vi "Main.vi"() -> ()   [LabVIEW 2020]
doc: "Cet exemple de projet Mesure continue est basé sur le modèle Gestionnaire de messages dans une file d'attente.\n\nLa boucle de gestion d'événements génère des messages en fonction des actions sur l'interface utilisateur.\n\nLa boucle de gestion de messages traite les messages générés par la boucle de gestion d'événements ou par d'autres messages. Il y a aussi des sous-VIs de boucle de gestion de messages d'acquisition et d'enregistrement, ainsi qu'une boucle de mise à jour du graphe déroulant."
uses:
  Settings/Settings.ctl
  Acquisition/Hardware Configuration.ctl
  Acquisition/Signal Type.ctl
  Logging/Logging Configuration.ctl
  controls/UI Data.ctl
  controls/UI State.ctl
  support/Message Queue/Enqueue Message (Single).vi
  support/Message Queue/Enqueue Message (Array).vi
  <vilib>/Utility/error.llb/Error Cluster From Error Code.vi
  <vilib>/ErrorRing/Error Ring.xnode
  Acquisition/Acquisition.lvlib
  Logging/Logging.lvlib
  Settings/Settings.lvlib
  support/User Event - Stop/User Event - Stop.lvlib
  support/Message Queue/Message Queue.lvlib
  Settings/Settings Dialog.vi
panel:
  in  "Panneaux":T1(tab)
  in  "Param status":bool
  out "Données":waveform(dbl)[](graph)
  out "État":string
  in  "Quitter":bool
  in  "Arrêter":bool
  in  "Démarrer":bool
  in  "Paramètres":bool
  out "Valeur des thermistantes 2":dbl[](array[numeric])
  out "Valeur des thermistantes":dbl[](array[numeric])
  # "TODO:\n\n- Mettre le port des paramètres pour connection\n- Faire entrer les param dans la boucle d'affichage\n- Valider l'enregistrement  du data\n- Faire sous-vi ordre 0\n- Faire sous-vi ordre 1"
  # "MAPA Tech"
  # "MAPA Tech"
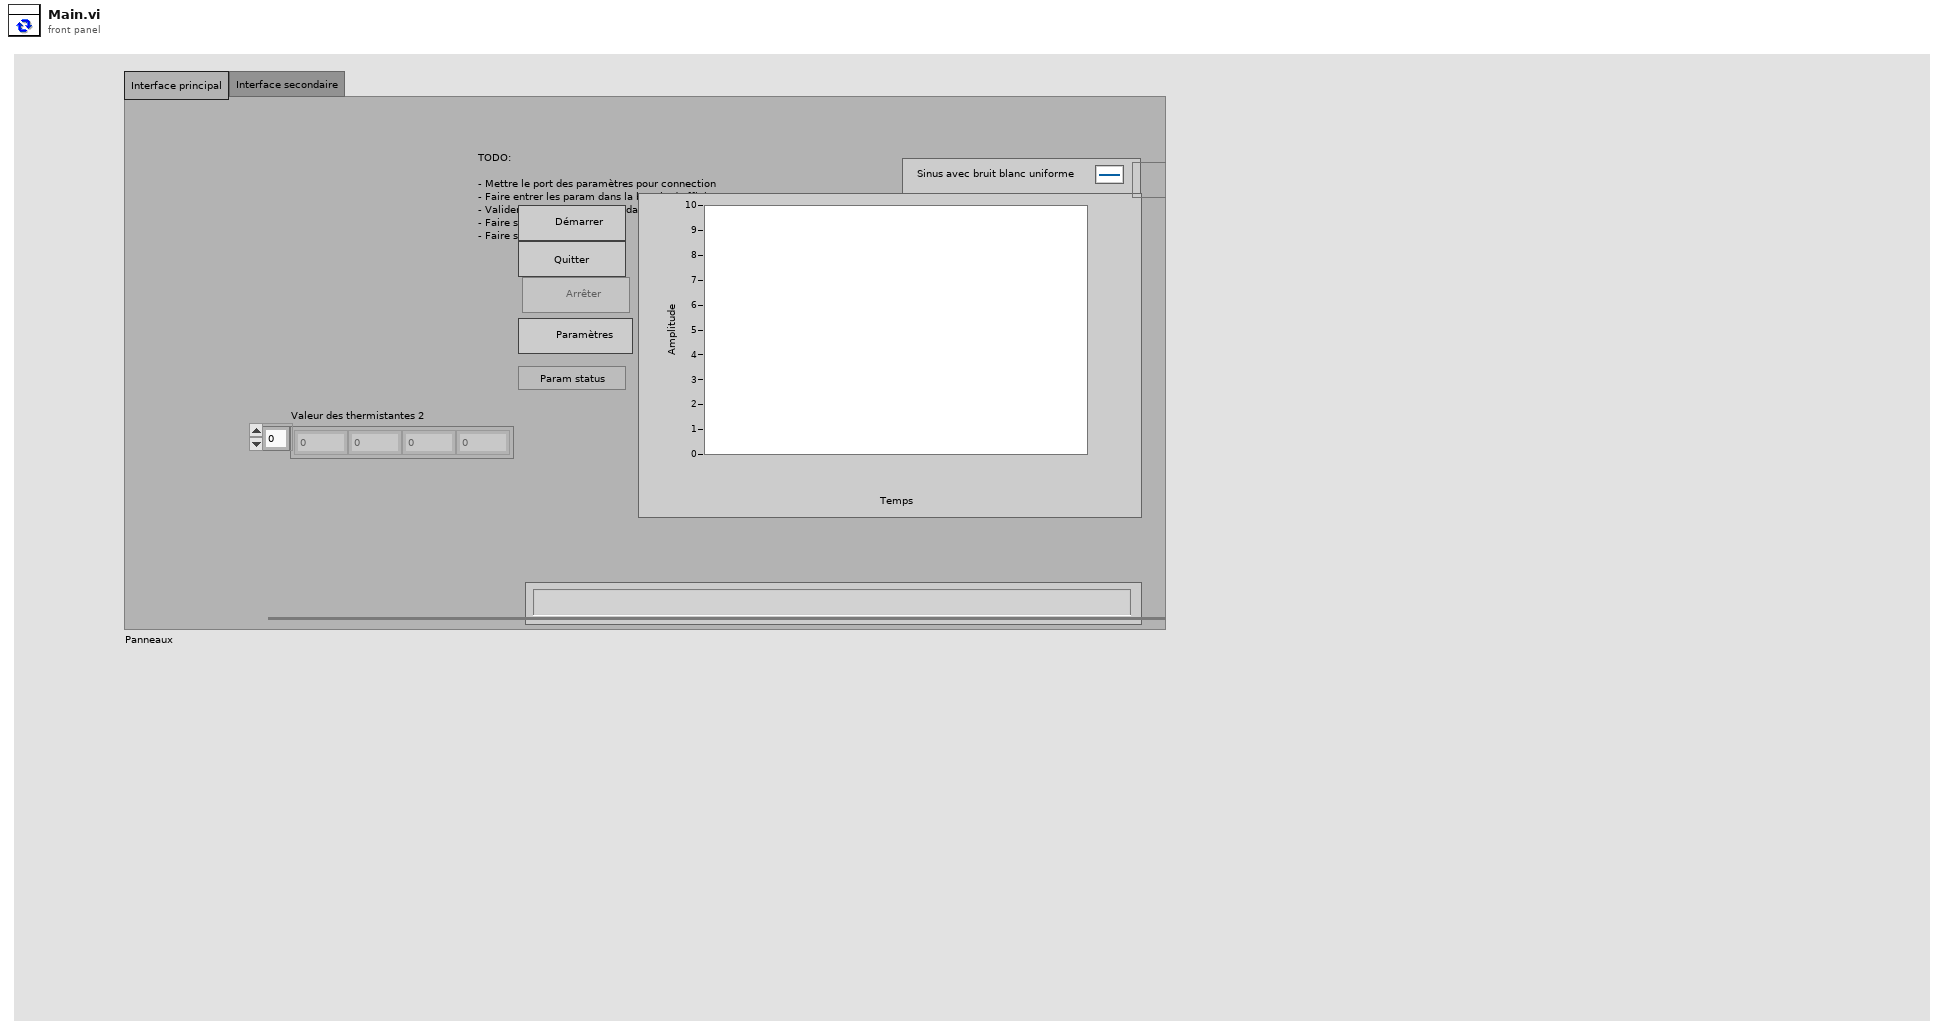
[diagram p1: front panel]
types:
  T1 = enum32{"Interface principal", "Interface secondaire"}
  T2 = typedef "UI State.ctl" = enum16{"Idle", "Acquiring and Logging", "Waiting for Exit", "Waiting for Exit (Acq Stopped)", "Waiting for Exit (Log Stopped)", "Waiting for Stop", "Waiting for Stop (Acq Stopped)", "Waiting for Stop (Log Stopped)"}
  T3 = typedef "UI Data.ctl" = cluster{"Réf. de Démarrer":refnum<vi>, "Réf. d'Arrêter":refnum<vi>, "Réf. de Paramètres":refnum<vi>, "Réf. de Quitter":refnum<vi>, "Réf. d'état":refnum<vi>, "Réf. de données":refnum<vi>, "Ref. Moyennage sélectionneur":refnum<vi>, "Ref. Param status":refnum<vi>}
  T4 = typedef "Settings.lvlib/Settings.ctl" = cluster{"Configuration du matériel":T5, "Configuration de l'enregistrement":T7, "Mode de longueur d'onde":cluster{"Choix du mode":bool, "Commande numérique":dbl}, "périphérique":cluster{"Nom du périphérique":tag}}
  T5 = typedef "Acquisition.lvlib/Hardware Configuration.ctl" = cluster{"Refnum de matériel <À remplacer>":string, "Type de signal <À remplacer>":T6}
  T6 = typedef "Acquisition.lvlib/Signal Type.ctl" = enum16{"Sine Wave", "Square with Noise", "Signal triangulaire", "Simulation DAQ"}
  T7 = typedef "Logging.lvlib/Logging Configuration.ctl" = cluster{"Chemin de base du fichier journal":path, "Référence de fichier TDMS":refnum<k34>}
  T8 = cluster{"état":bool, "code":i32, "source":string}
  T9 = typedef "Message Queue.lvlib/All Message Queues.ctl" = cluster{"IU":refnum<queue>, "Acquisition":refnum<queue>, "Enregistrement":refnum<queue>}
  T10 = cluster{"Choix du mode":bool, "Commande numérique":dbl}
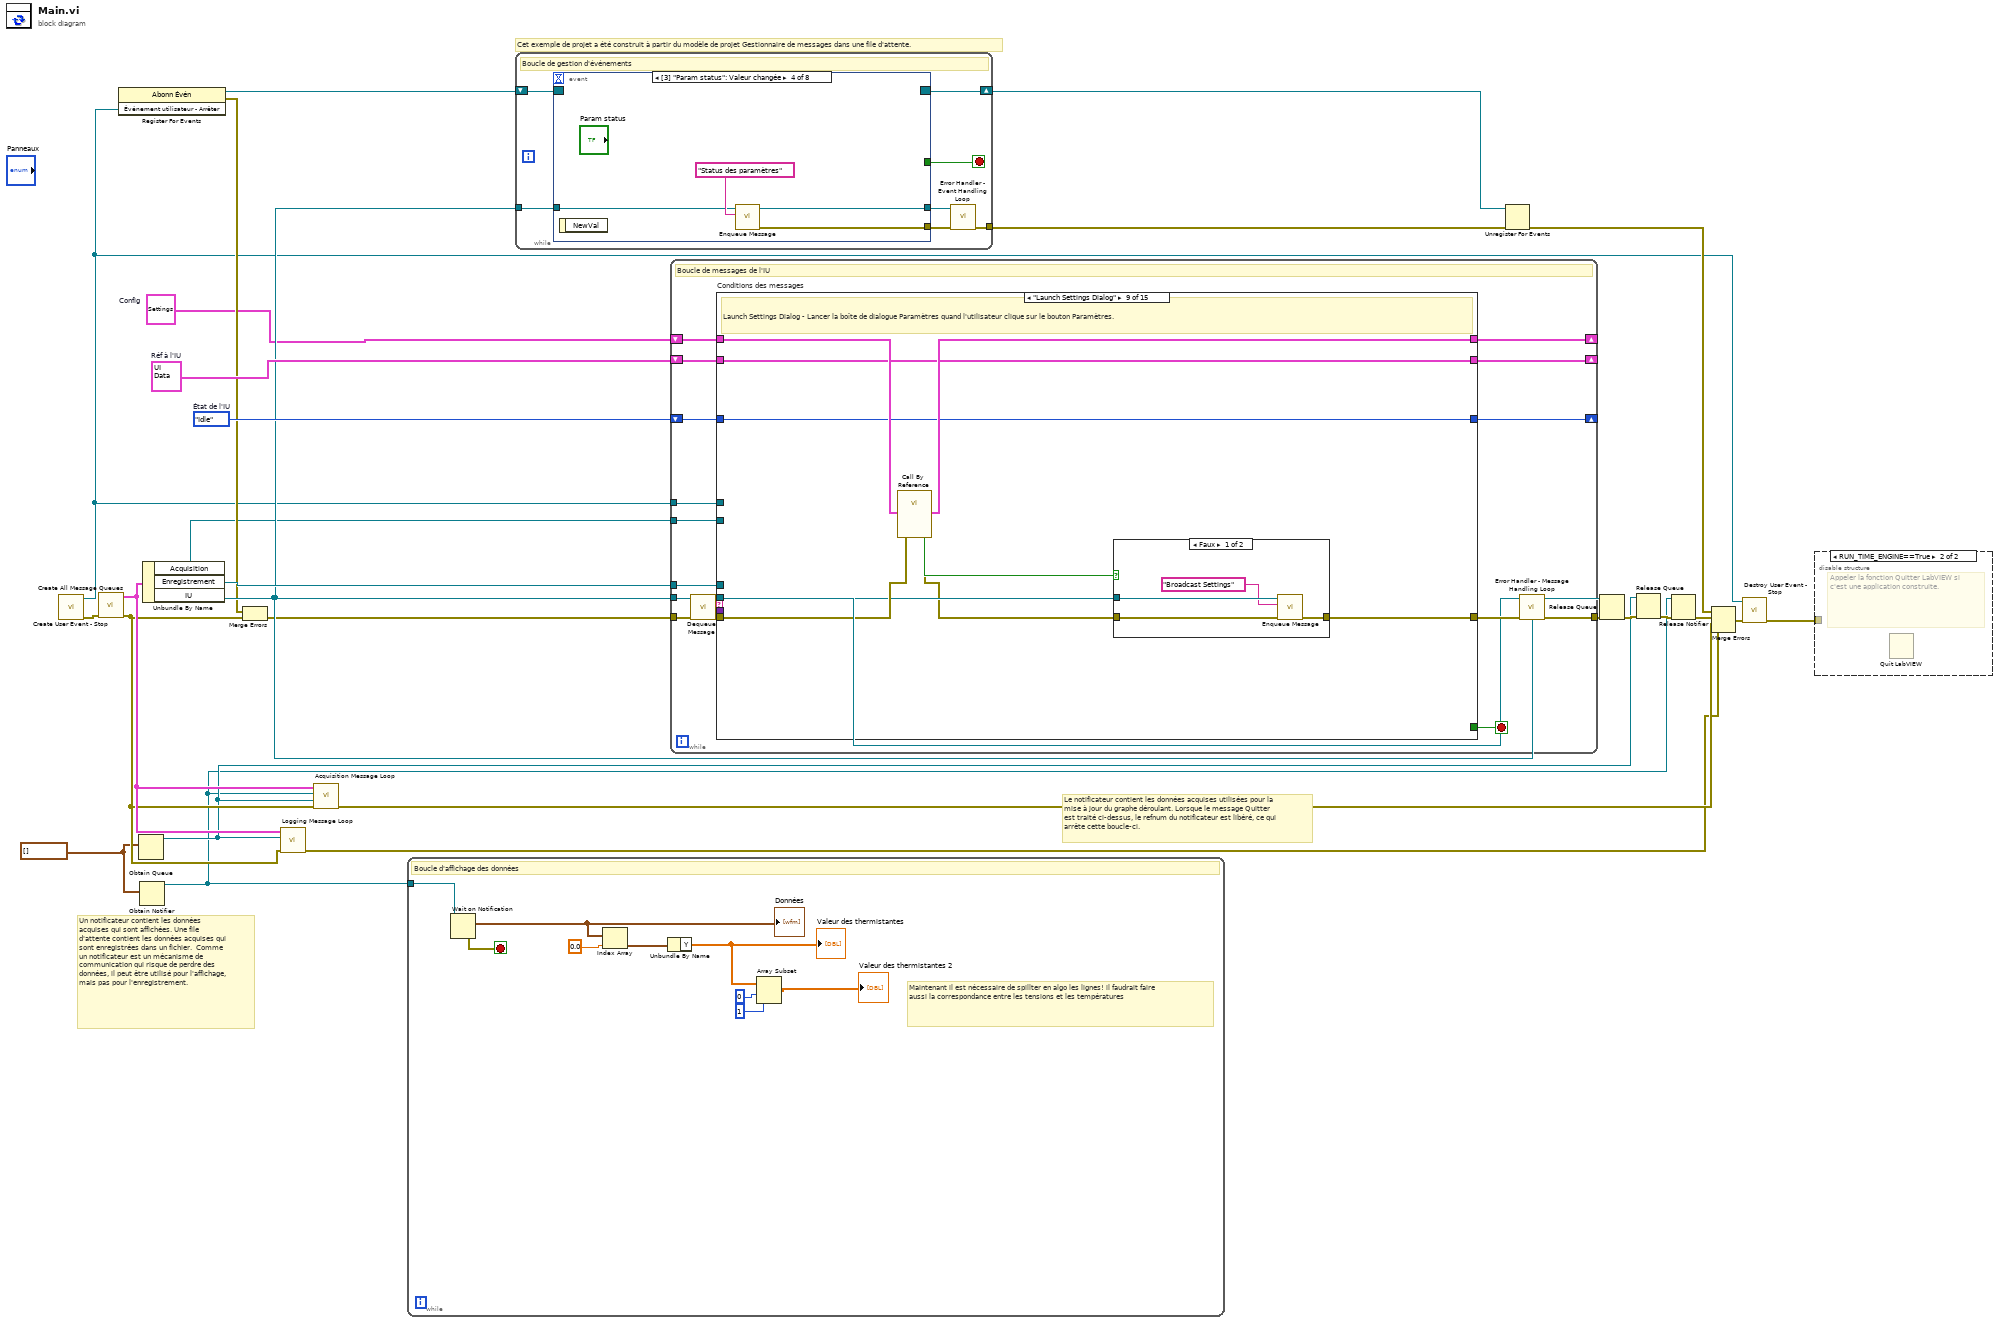
[diagram p0: block diagram]
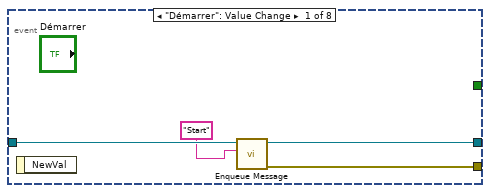
[diagram p3: hidden frame]
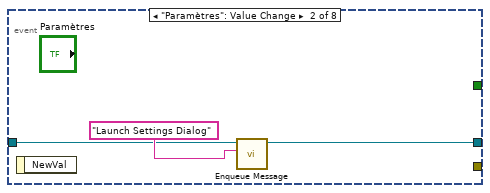
[diagram p4: hidden frame]
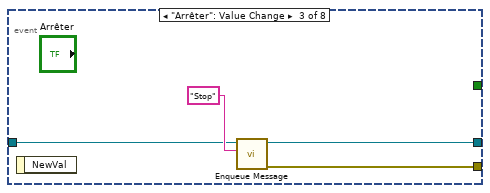
[diagram p5: hidden frame]
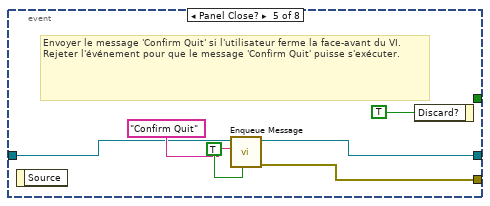
[diagram p6: hidden frame]
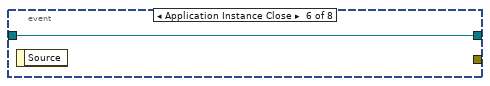
[diagram p7: hidden frame]
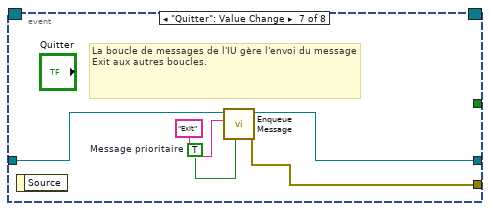
[diagram p8: hidden frame]
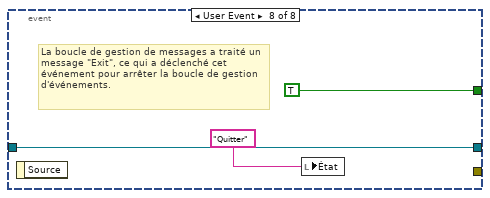
[diagram p9: hidden frame]
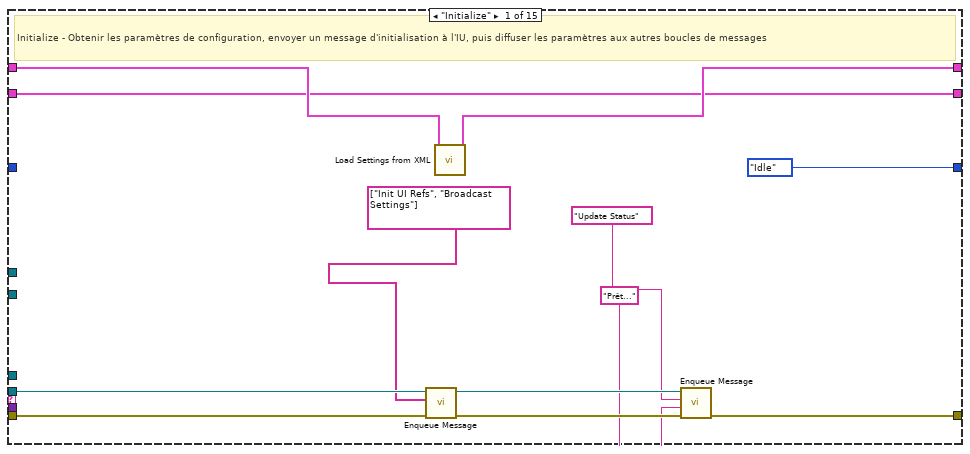
[diagram p10: hidden frame]
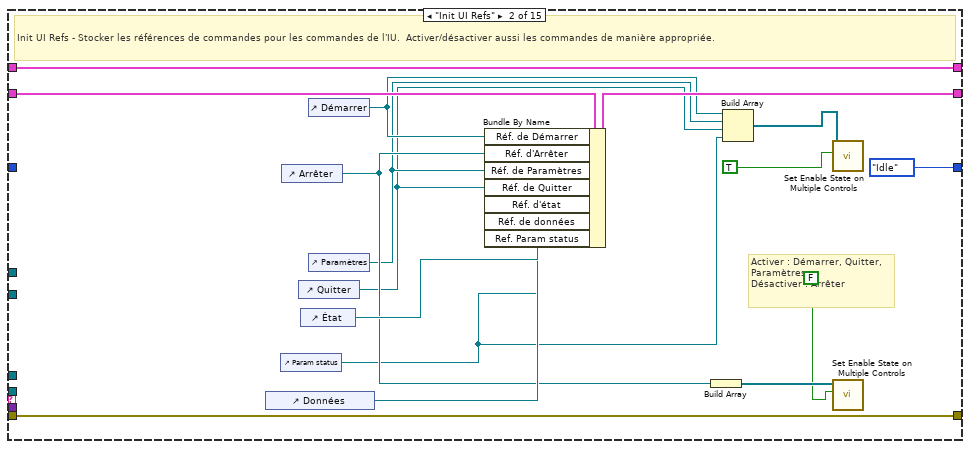
[diagram p11: hidden frame]
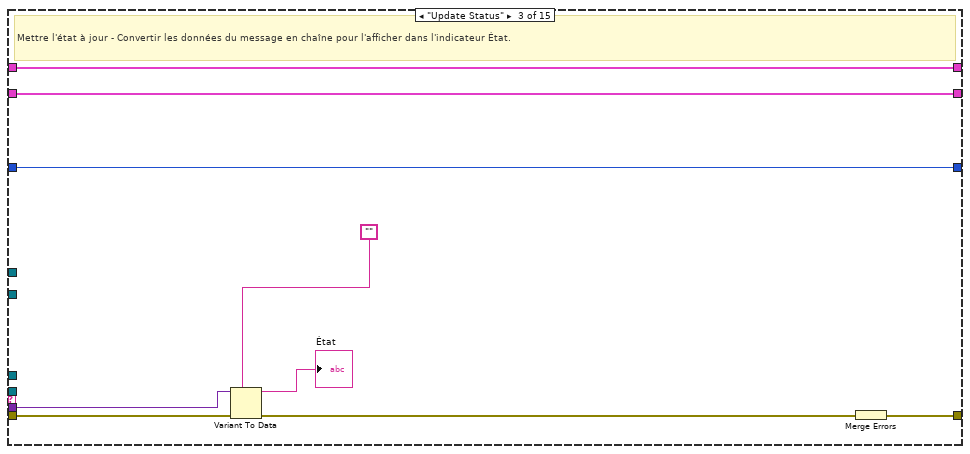
[diagram p12: hidden frame]
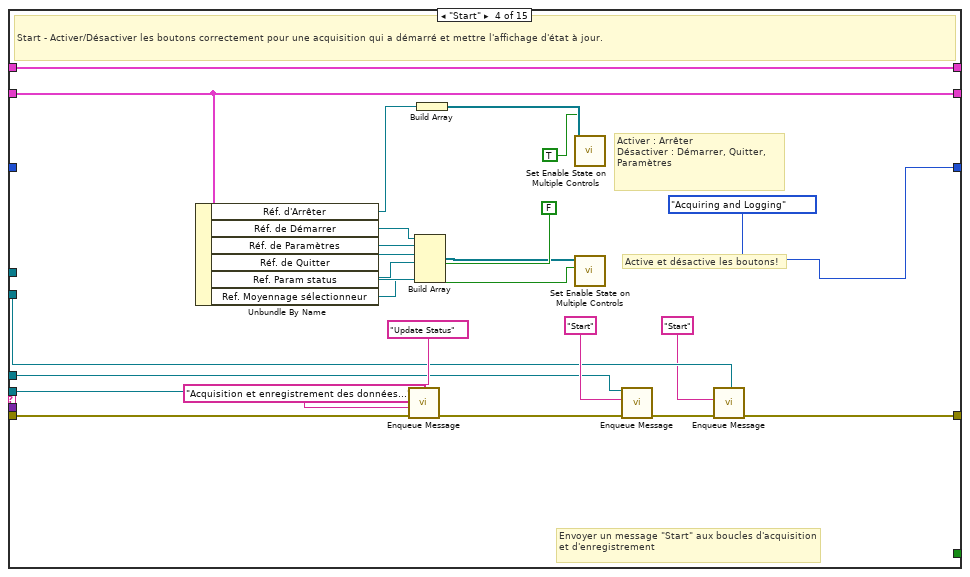
[diagram p13: hidden frame]
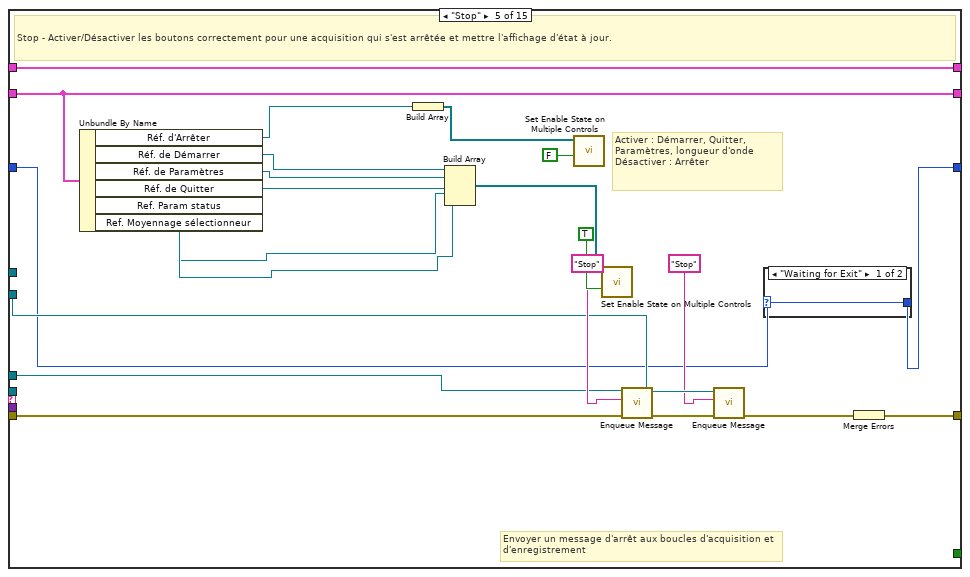
[diagram p14: hidden frame]
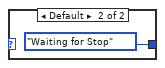
[diagram p15: hidden frame]
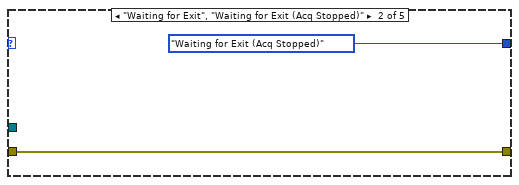
[diagram p17: hidden frame]
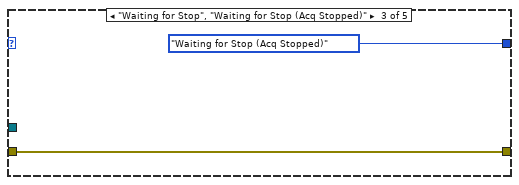
[diagram p18: hidden frame]
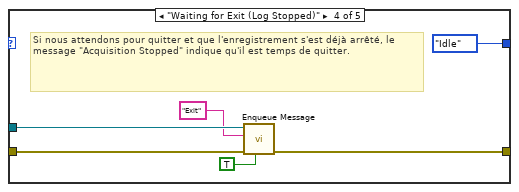
[diagram p19: hidden frame]
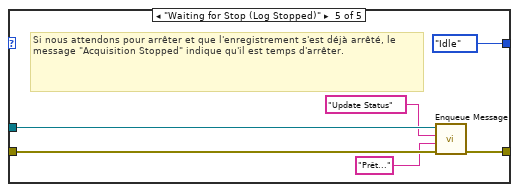
[diagram p20: hidden frame]
diagram:
  w16 = UI_State."Idle"  # État de l'IU
  w2 = waveform(dbl)[] []
  w18 = T3 {"Réf. de Démarrer"=refnum, "Réf. d'Arrêter"=refnum, "Réf. de Paramètres"=refnum, "Réf. de Quitter"=refnum, "Réf. d'état"=refnum, "Réf. de données"=refnum, "Ref. Moyennage sélectionneur"=refnum, "Ref. Param status"=refnum}  # Réf à l'IU
  w1 = T4 {"Configuration du matériel"={"Refnum de matériel <À remplacer>"="", "Type de signal <À remplacer>"=enum."Simulation DAQ"}, "Configuration de l'enregistrement"={"Chemin de base du fichier journal"=path "", "Référence de fichier TDMS"=refnum}, "Mode de longueur d'onde"={"Choix du mode"=TRUE, "Commande numérique"=15.0}, "périphérique"={"Nom du périphérique"="Dev1"}}  # Config
  # "Cet exemple de projet a été construit à partir du modèle de projet Gestionnaire de messages dans une file d'attente."
  # "Un notificateur contient les données acquises qui sont affichées. Une file d'attente contient les données acquises qui sont enregistrées dans un fichier.  Comme un notificateur est un mécanisme de communication qui risque de perdre des données, il peut être utilisé pour l'affichage, mais pas pour l'enregistrement."
  # "Le notificateur contient les données acquises utilisées pour la mise à jour du graphe déroulant. Lorsque le message Quitter est traité ci-dessus, le refnum du notificateur est libéré, ce qui arrête cette boucle-ci."
  n1 = call "Create User Event - Stop.vi"() -> ("error out"=w24:T8, "Événement utilisateur - Arrêter"=w3:refnum<user-event>)  [unwired: 10 in]
  n2 = call "Create All Message Queues.vi"("error in (no error)"=w24) -> ("error out"=w21:T8, "Files d'attente de messages en sortie"=w23:T9)  [unwired: 9 in]
  n3 = register-events(w3) -> (reference out=w7:refnum<event-registration>, error out=w5:errorcluster)  [unwired: 2 in]
  n4 = Obtain Queue(element data type=w2) -> (queue out=w9:refnum<queue>)  [unwired: 4 in, 2 out]
  n5 = Obtain Notifier(notification data type=w2) -> (notifier out=w8:refnum<notifier>)  [unwired: 3 in, 2 out]
  n6 = Unbundle By Name(w23) -> ("Acquisition"=w4:refnum<queue>, "Enregistrement"=w17:refnum<queue>, "IU"=w14:refnum<queue>)
  n7 = Merge Errors(w5, w21) -> (w6:errorcluster)
  n8 = call "Logging Message Loop.vi"("error in (no error)"=w21, "File d'attente de données"=w9, "Files d'attente de messages"=w23) -> ("error out"=w22:T8)  [unwired: 8 in]
  n9 = call "Acquisition Message Loop.vi"("error in (no error)"=w21, "File d'attente de données"=w9, "Notificateur de données"=w8, "Files d'attente de messages"=w23) -> ("error out"=w25:T8)  [unwired: 7 in]
  n10 = while "Data Display Loop" {
    tunnel: w8 -> [w35]
    stop <- w36 stop-if-true
    # "Maintenant il est nécessaire de spillter en algo les lignes! il faudrait faire aussi la correspondance entre les tensions et les températures"
    # "Boucle d'affichage des données"
    n11 = Wait on Notification(notifier=w35) -> (notification=w33:waveform(dbl)[], error out=w36:errorcluster)  [unwired: 3 in, 2 out]
    "Données" <- w33
    n12 = Index Array(array=w33, index=0.0) -> (element=w32:waveform(dbl))
    n13 = Unbundle By Name(w32) -> ("Y"=w28:dbl[])
    "Valeur des thermistantes" <- w28
    n14 = Array Subset(array=w28, index=0 ("indice"), length=1 ("longueur")) -> (→"Valeur des thermistantes 2":dbl[])
  }
  n15 = while {
    tunnel: w14 -> [w42]
    tunnel: [w39] -> w26
    shift-right: [w41] -> w19
    shift-left: w7 -> [w43]
    stop <- w40 stop-if-true
    # "Boucle de gestion d'événements"
    n16 = event shown="[3] \"Param status\": Valeur changée" {
      selector: w43 -> [_ _ _ _ _ _ _ _]
      dyn-events: [_ _ _ _ _ _ _ _] -> w41
      timeout: _ -> [_ _ _ _ _ _ _ _]
      tunnel: [_ _ _ _ _ _ _ TRUE ("Discard?")] -> w40
      tunnel: w42 -> [w47 w49 w53 w57 w62 w65 w67 w71]
      tunnel: [w45 _ w52 w56 w60 _ w70 _] -> w38
      tunnel: [w44 w48 w51 w55 w61 w65 w66 w71] -> w37
      event "Démarrer": Value Change {
        n17 = event-data() -> ()  [unwired: 1 in, 1 out]
        n18 = call-poly "Enqueue Message.vi"("Message"="Start", "File d'attente de messages"=w47) -> ("error out"=w45:T8, "File d'attente de message dup."=w44:refnum<queue>)  [unwired: 8 in]
      }
      event "Paramètres": Value Change {
        n19 = event-data() -> ()  [unwired: 1 in, 1 out]
        n20 = call-poly "Enqueue Message.vi"("Message"="Launch Settings Dialog", "File d'attente de messages"=w49) -> ("File d'attente de message dup."=w48:refnum<queue>)  [unwired: 8 in, 1 out]
      }
      event "Arrêter": Value Change {
        n21 = event-data() -> ()  [unwired: 1 in, 1 out]
        n22 = call-poly "Enqueue Message.vi"("Message"="Stop", "File d'attente de messages"=w53) -> ("error out"=w52:T8, "File d'attente de message dup."=w51:refnum<queue>)  [unwired: 8 in]
      }
      event "Param status": Value Change {
        n23 = event-data() -> ()  [unwired: 1 in, 1 out]
        n24 = call-poly "Enqueue Message.vi"("Message"="Status des paramètres", "File d'attente de messages"=w57) -> ("error out"=w56:T8, "File d'attente de message dup."=w55:refnum<queue>)  [unwired: 8 in]
      }
      event Panel Close? {
        # "Envoyer le message 'Confirm Quit' si l'utilisateur ferme la face-avant du VI. Rejeter l'événement pour que le message 'Confirm Quit' puisse s'exécuter."
        n25 = event-data() -> ()  [unwired: 1 in, 1 out]
        n26 = call-poly "Enqueue Message.vi"("Message prioritaire ? (F)"=TRUE ("Priority Message? (F)"), "Message"="Confirm Quit", "File d'attente de messages"=w62) -> ("error out"=w60:T8, "File d'attente de message dup."=w61:refnum<queue>)  [unwired: 7 in]
        n27 = event-data ("Event Filter Node")("Discard?"=TRUE) -> ()  [unwired: 1 in, 1 out]
      }
      event Application Instance Close {
        n28 = event-data() -> ()  [unwired: 1 in, 1 out]
      }
      event "Quitter": Value Change {
        w68 = TRUE  # Message prioritaire
        # "La boucle de messages de l'IU gère l'envoi du message Exit aux autres boucles."
        n29 = event-data() -> ()  [unwired: 1 in, 1 out]
        n30 = call-poly "Enqueue Message.vi"("Message prioritaire ? (F)"=w68, "Message"="Exit", "File d'attente de messages"=w67) -> ("error out"=w70:T8, "File d'attente de message dup."=w66:refnum<queue>)  [unwired: 7 in]
      }
      event User Event {
        # "La boucle de gestion de messages a traité un message \"Exit\", ce qui a déclenché cet événement pour arrêter la boucle de gestion d'événements."
        n31 = event-data() -> ()  [unwired: 1 in, 1 out]
        n32 = local write "État"("Quitter" ("Exit String")) -> ()
      }
    }
    n33 = call "Error Handler - Event Handling Loop.vi"("error in (no error)"=w38, "File d'attente de messages"=w37) -> ("erreur en entrée dup."=w39:T8)  [unwired: 8 in, 1 out]
  }
  n34 = while {
    tunnel: w14 -> [w85]
    tunnel: w3 -> [w90]
    shift-right: [w84] -> _
    shift-left: w1 -> [w83]
    shift-right: [w81] -> _
    shift-left: w18 -> [w82]
    tunnel: w4 -> [w80]
    tunnel: w17 -> [w79]
    shift-right: [w74] -> _
    shift-left: w16 -> [w75]
    tunnel: w6 -> [w89]
    tunnel: [w78] -> w27
    stop <- w91 stop-if-true
    # "Boucle de messages de l'IU"
    n35 = call "Dequeue Message.vi"("error in (no error)"=w89, "File d'attente de messages"=w85) -> ("error out"=w88:T8, "Données de message"=w86:variant, "Message"=w87:string, "File d'attente de message dup."=w76:refnum<queue>)  [unwired: 6 in]
    n36 = case "Conditions des messages" shown="\"Launch Settings Dialog\"" w87 {
      selector: w87 -> [_ _ _ _ _ _ _ _ _ _ _ _ _ _ w331]
      tunnel: w76 -> [w95 _ _ w152 _ w179 w204 _ w246 _ w267 _ _ w318 _]
      tunnel: w88 -> [w94 w119 w127 w151 w173 w180 w205 w234 w248 w255 w266 w295 w312 w322 _]
      tunnel: [w99 w119 w128 w138 w174 w177 w202 w240 w241 w258 w265 w305 w311 w321 w330] -> w77
      tunnel: [_ _ _ _ _ _ _ _ _ _ _ TRUE _ _ _] -> w91
      tunnel: w86 -> [_ _ w126 _ _ _ _ _ _ w259 _ w293 _ _ _]
      tunnel: w90 -> [_ _ _ _ _ _ _ _ _ _ _ w306 _ _ _]
      tunnel: [w102 w118 w122 w150 w172 w183 w208 w238 w245 w263 w270 w304 w310 w316 w334] -> w84
      tunnel: w83 -> [w103 w118 w122 w150 w172 w183 w208 w238 w249 w263 w270 w304 w310 w316 w334]
      tunnel: w82 -> [w96 w117 w121 w147 w171 w182 w207 w233 w243 w262 w269 w303 w309 w320 w333]
      tunnel: [w96 w114 w121 w147 w171 w182 w207 w233 w243 w262 w269 w303 w309 w320 w333] -> w81
      tunnel: w80 -> [_ _ _ w137 w164 _ _ w232 _ _ _ w302 _ _ _]
      tunnel: w79 -> [_ _ _ w140 w167 _ _ w227 _ _ _ w301 _ _ _]
      tunnel: w75 -> [_ _ w120 _ w161 w181 w206 w231 w242 w257 w268 _ w308 _ w332]
      tunnel: [UI_State."Idle" ("UI State") UI_State."Idle" ("UI State") w120 UI_State."Acquiring and Logging" ("UI State") w162 w178 w203 w231 w242 w257 w264 UI_State."Idle" ("UI State") w308 UI_State."Acquiring and Logging" ("UI State") w332] -> w74
      frame "Initialize" {
        # "Initialize - Obtenir les paramètres de configuration, envoyer un message d'initialisation à l'IU, puis diffuser les paramètres aux autres boucles de messages"
        n37 = call-poly "Enqueue Message.vi"("error in (no error)"=w94, "Tableau de messages"=string[] ["Init UI Refs", "Broadcast Settings"], "File d'attente de messages"=w95) -> ("error out"=w101:T8, "File d'attente de message dup."=w100:refnum<queue>)  [unwired: 7 in]
        n38 = call "Load Settings from XML.vi"("Paramètres en entrée"=w103) -> ("Paramètres en sortie"=w102:T4)  [unwired: 9 in, 1 out]
        n39 = call-poly "Enqueue Message.vi"("error in (no error)"=w101, "Données de message"="Prêt..." ("Ready..."), "Message"="Update Status", "File d'attente de messages"=w100) -> ("error out"=w99:T8)  [unwired: 6 in, 1 out]
      }
      frame "Init UI Refs" {
        # "Activer : Démarrer, Quitter, Paramètres\nDésactiver : Arrêter"
        # "Init UI Refs - Stocker les références de commandes pour les commandes de l'IU.  Activer/désactiver aussi les commandes de manière appropriée."
        n40 = control-ref of="Données"() -> (w115:refnum<vi>)
        n41 = control-ref of="Param status"() -> (w104:refnum<vi>)
        n42 = control-ref of="Arrêter"() -> (w109:refnum<vi>)
        n43 = control-ref of="Quitter"() -> (w106:refnum<vi>)
        n44 = control-ref of="État"() -> (w116:refnum<vi>)
        n45 = control-ref of="Démarrer"() -> (w108:refnum<vi>)
        n46 = control-ref of="Paramètres"() -> (w107:refnum<vi>)
        n47 = Bundle By Name(cluster=w117, "Réf. de Démarrer"=w108, "Réf. d'Arrêter"=w109, "Réf. de Paramètres"=w107, "Réf. de Quitter"=w106, "Réf. d'état"=w116, "Réf. de données"=w115, "Ref. Param status"=w104) -> (w114:T3)
        n48 = Build Array(w109) -> (w111:refnum<vi>[])
        n49 = Build Array(w108, w107, w106, w104) -> (w112:refnum<vi>[])
        n50 = call "Set Enable State on Multiple Controls.vi"("Activé ?"=TRUE ("Enable?"), "Commandes"=w112) -> ()  [unwired: 10 in]
        n51 = call "Set Enable State on Multiple Controls.vi"("Activé ?"=FALSE ("Enable?"), "Commandes"=w111) -> ()  [unwired: 10 in]
      }
      frame "Update Status" {
        # "Mettre l'état à jour - Convertir les données du message en chaîne pour l'afficher dans l'indicateur État."
        n52 = Variant To Data(error in=w127, type="" ("Empty String Constant"), Variant=w126) -> (data=→"État":string, error out=w124:errorcluster)
        n53 = Merge Errors(w124) -> (w128:errorcluster)
      }
      frame "Start" {
        # "Active et désactive les boutons!"
        # "Envoyer un message \"Start\" aux boucles d'acquisition et d'enregistrement"
        # "Activer : Arrêter\nDésactiver : Démarrer, Quitter, Paramètres"
        # "Start - Activer/Désactiver les boutons correctement pour une acquisition qui a démarré et mettre l'affichage d'état à jour."
        n54 = Unbundle By Name(w147) -> ("Réf. d'Arrêter"=w129:refnum<vi>, "Réf. de Démarrer"=w130:refnum<vi>, "Réf. de Paramètres"=w131:refnum<vi>, "Réf. de Quitter"=w134:refnum<vi>, "Ref. Param status"=w133:refnum<vi>, "Ref. Moyennage sélectionneur"=w132:refnum<vi>)
        n55 = call-poly "Enqueue Message.vi"("error in (no error)"=w151, "Données de message"="Acquisition et enregistrement des données..." ("Acquiring and Logging..."), "Message"="Update Status", "File d'attente de messages"=w152) -> ("error out"=w142:T8)  [unwired: 6 in, 1 out]
        n56 = Build Array(w130, w131, w131, w134, w133, w132) -> (w145:refnum<vi>[])
        n57 = Build Array(w129) -> (w144:refnum<vi>[])
        n58 = call "Set Enable State on Multiple Controls.vi"("Activé ?"=TRUE ("Enable?"), "Commandes"=w144) -> ()  [unwired: 10 in]
        n59 = call "Set Enable State on Multiple Controls.vi"("Activé ?"=FALSE ("Enable?"), "Commandes"=w145) -> ()  [unwired: 10 in]
        n60 = call-poly "Enqueue Message.vi"("error in (no error)"=w142, "Message"="Start", "File d'attente de messages"=w140) -> ("error out"=w139:T8)  [unwired: 7 in, 1 out]
        n61 = call-poly "Enqueue Message.vi"("error in (no error)"=w139, "Message"="Start", "File d'attente de messages"=w137) -> ("error out"=w138:T8)  [unwired: 7 in, 1 out]
      }
      frame "Stop" {
        # "Envoyer un message d'arrêt aux boucles d'acquisition et d'enregistrement"
        # "Activer : Démarrer, Quitter, Paramètres, longueur d'onde\nDésactiver : Arrêter"
        # "Stop - Activer/Désactiver les boutons correctement pour une acquisition qui s'est arrêtée et mettre l'affichage d'état à jour."
        n62 = Unbundle By Name(w171) -> ("Réf. d'Arrêter"=w153:refnum<vi>, "Réf. de Démarrer"=w154:refnum<vi>, "Réf. de Paramètres"=w155:refnum<vi>, "Réf. de Quitter"=w156:refnum<vi>, "Ref. Param status"=w157:refnum<vi>, "Ref. Moyennage sélectionneur"=w158:refnum<vi>)
        n63 = Build Array(w153) -> (w159:refnum<vi>[])
        n64 = Build Array(w154, w155, w156, w157, w158) -> (w160:refnum<vi>[])
        n65 = call "Set Enable State on Multiple Controls.vi"("Activé ?"=FALSE ("Enable?"), "Commandes"=w159) -> ()  [unwired: 10 in]
        n66 = call "Set Enable State on Multiple Controls.vi"("Activé ?"=TRUE ("Enable?"), "Commandes"=w160) -> ()  [unwired: 10 in]
        n67 = call-poly "Enqueue Message.vi"("error in (no error)"=w173, "Message"="Stop", "File d'attente de messages"=w167) -> ("error out"=w166:T8)  [unwired: 7 in, 1 out]
        n68 = call-poly "Enqueue Message.vi"("error in (no error)"=w166, "Message"="Stop", "File d'attente de messages"=w164) -> ("error out"=w165:T8)  [unwired: 7 in, 1 out]
        n69 = case shown="\"Waiting for Exit\"" w161 {
          selector: w161 -> [w175 _]
          tunnel: [w175 UI_State."Waiting for Stop" ("UI State")] -> w162
          frame "Waiting for Exit" {
          }
          frame Default {
          }
        }
        n70 = Merge Errors(w165) -> (w174:errorcluster)
      }
      frame "Acquisition Stopped" {
        # "Logique déterminant quelle action entreprendre quand l'acquisition s'est arrêtée."
        n71 = case shown="Par défaut" w181 {
          selector: w181 -> [w185 _ _ _ _]
          tunnel: w180 -> [w184 w187 w189 w195 w201]
          tunnel: w179 -> [_ _ _ w193 w198]
          tunnel: [w185 UI_State."Waiting for Exit (Acq Stopped)" ("UI State") UI_State."Waiting for Stop (Acq Stopped)" ("UI State") UI_State."Idle" ("UI State") UI_State."Idle" ("UI State")] -> w178
          tunnel: [w184 w187 w189 w194 w199] -> w177
          frame Default {
          }
          frame "Waiting for Exit", "Waiting for Exit (Acq Stopped)" {
          }
          frame "Waiting for Stop", "Waiting for Stop (Acq Stopped)" {
          }
          frame "Waiting for Exit (Log Stopped)" {
            # "Si nous attendons pour quitter et que l'enregistrement s'est déjà arrêté, le message \"Acquisition Stopped\" indique qu'il est temps de quitter."
            n72 = call-poly "Enqueue Message.vi"("Message prioritaire ? (F)"=TRUE ("Priority Message? (F)"), "error in (no error)"=w195, "Message"="Exit", "File d'attente de messages"=w193) -> ("error out"=w194:T8)  [unwired: 6 in, 1 out]
          }
          frame "Waiting for Stop (Log Stopped)" {
            # "Si nous attendons pour arrêter et que l'enregistrement s'est déjà arrêté, le message \"Acquisition Stopped\" indique qu'il est temps d'arrêter."
            n73 = call-poly "Enqueue Message.vi"("error in (no error)"=w201, "Données de message"="Prêt..." ("Ready..."), "Message"="Update Status", "File d'attente de messages"=w198) -> ("error out"=w199:T8)  [unwired: 6 in, 1 out]
          }
        }
      }
      frame "Logging Stopped" {
        # "Logique déterminant quelle action entreprendre quand l'enregistrement s'est arrêté."
        n74 = case shown="\"Waiting for Stop (Acq Stopped)\"" w206 {
          selector: w206 -> [w210 _ _ _ _]
          tunnel: w205 -> [w209 w212 w214 w220 w223]
          tunnel: w204 -> [_ _ _ w218 w222]
          tunnel: [w210 UI_State."Waiting for Exit (Log Stopped)" ("UI State") UI_State."Waiting for Stop (Log Stopped)" ("UI State") UI_State."Idle" ("UI State") UI_State."Idle" ("UI State")] -> w203
          tunnel: [w209 w212 w214 w219 w221] -> w202
          frame Default {
          }
          frame "Waiting for Exit", "Waiting for Exit (Log Stopped)" {
          }
          frame "Waiting for Stop", "Waiting for Stop (Log Stopped)" {
          }
          frame "Waiting for Exit (Acq Stopped)" {
            # "Si nous attendons pour quitter et que l'acquisition s'est déjà arrêtée, le message \"Logging Stopped\" indique qu'il est temps de quitter."
            n75 = call-poly "Enqueue Message.vi"("Message prioritaire ? (F)"=TRUE ("Priority Message? (F)"), "error in (no error)"=w220, "Message"="Exit", "File d'attente de messages"=w218) -> ("error out"=w219:T8)  [unwired: 6 in, 1 out]
          }
          frame "Waiting for Stop (Acq Stopped)" {
            # "Si nous attendons pour arrêter et que l'acquisition s'est déjà arrêtée, le message \"Logging Stopped\" indique qu'il est temps d'arrêter."
            n76 = call-poly "Enqueue Message.vi"("error in (no error)"=w223, "Données de message"="Prêt..." ("Ready..."), "Message"="Update Status", "File d'attente de messages"=w222) -> ("error out"=w221:T8)  [unwired: 6 in, 1 out]
          }
        }
      }
      frame "Broadcast settings" {
        w228 = "Update Settings" ("Message")
        # "Broadcast settings - Envoyer le message 'Update Settings' aux boucles de messages d'enregistrement et d'acquisition."
        n77 = Unbundle By Name(w238) -> ("Configuration du matériel"=w237:T5, "Configuration de l'enregistrement"=w236:T7, "Mode de longueur d'onde"=w230:T10)
        n78 = call-poly "Enqueue Message.vi"("Données de message"=w237, "Message"=w228, "File d'attente de messages"=w232) -> ("error out"=w239:T8)  [unwired: 7 in, 1 out]
        n79 = call-poly "Enqueue Message.vi"("Données de message"=w230, "Message"=w228, "File d'attente de messages"=w227) -> ("error out"=w229:T8)  [unwired: 7 in, 1 out]
        n80 = call-poly "Enqueue Message.vi"("error in (no error)"=w239, "Données de message"=w236, "Message"=w228, "File d'attente de messages"=w227) -> ("error out"=w235:T8)  [unwired: 6 in, 1 out]
        n81 = Merge Errors(w229, w235, w234) -> (w240:errorcluster)
      }
      frame "Launch Settings Dialog" {
        # "Launch Settings Dialog - Lancer la boîte de dialogue Paramètres quand l'utilisateur clique sur le bouton Paramètres."
        n82 = call-by-ref "?"("error in (no error)"=w248, "Paramètres en entrée"=w249) -> ("error out"=w244:T8, "Annulation ?"=w247:bool, "Paramètres en sortie"=w245:T4)  [unwired: 8 in, 3 out]
        n83 = case shown="Faux" w247 {
          tunnel: w246 -> [w253 _]
          tunnel: w244 -> [w252 w254]
          tunnel: [w251 w254] -> w241
          frame False {
            n84 = call-poly "Enqueue Message.vi"("error in (no error)"=w252, "Message"="Broadcast Settings", "File d'attente de messages"=w253) -> ("error out"=w251:T8)  [unwired: 7 in, 1 out]
          }
          frame True {
          }
        }
      }
      frame "Error" {
        # "Error - Afficher une boîte de dialogue d'erreur. Ce message est envoyé par les VIs \"Error Handler\" à la fin de l'exécution de chaque boucle de cette application."
        n85 = Variant To Data(error in=w255, type=errorcluster {"status"=FALSE, "code"=0, "source"=""} ("error constant"), Variant=w259) -> (data=w256:errorcluster, error out=w260:errorcluster)
        n86 = call <vilib>:"Simple Error Handler.vi"("error in (no error)"=w256) -> ()  [unwired: 4 in, 5 out]
        n87 = Merge Errors(w260) -> (w258:errorcluster)
      }
      frame "Confirm Quit" {
        # "Confirm Quit - Message qui confirme si l'utilisateur voulait vraiment quitter l'application."
        n88 = case shown="\"Acquiring and Logging\"" w268 {
          tunnel: w267 -> [w276 w280]
          tunnel: w266 -> [w275 w279]
          tunnel: [w274 w278] -> w265
          tunnel: [UI_State."Idle" ("UI State") w277] -> w264
          frame Default {
            # "Si 'Confirm Quit' survient alors que le système est inactif, le message de confirmation est inutile."
            n89 = call-poly "Enqueue Message.vi"("Message prioritaire ? (F)"=TRUE ("Priority Message? (F)"), "error in (no error)"=w275, "Message"="Exit", "File d'attente de messages"=w276) -> ("error out"=w274:T8)  [unwired: 6 in, 1 out]
          }
          frame "Acquiring and Logging" {
            n90 = Two Button Dialog(message="Voulez-vous vraiment quitter en cours d'acquisition ?" ("Confirm Quit Message"), 1:"Non" ("No"), 2:"Oui" ("Yes")) -> (T button?=w281:bool)
            n91 = case shown="Vrai" w281 {
              tunnel: w280 -> [_ w290]
              tunnel: w279 -> [w286 w291]
              tunnel: [w286 w289] -> w278
              tunnel: [UI_State."Acquiring and Logging" ("UI State") UI_State."Waiting for Exit" ("UI State")] -> w277
              frame False {
                # "L'utilisateur ne voulait pas quitter."
              }
              frame True {
                n92 = call-poly "Enqueue Message.vi"("error in (no error)"=w291, "Message"="Stop", "File d'attente de messages"=w290) -> ("error out"=w289:T8)  [unwired: 7 in, 1 out]
              }
            }
          }
        }
      }
      frame "Exit" {
        w297 = TRUE ("Priority Message? (F)")
        w298 = "Exit" ("Message")
        # "Afficher une boîte de dialogue d'erreur si 'Exit' a été appelé suite à une erreur."
        # "Arrêter le VI"
        # "Exit - Envoyer des messages Exit aux boucles d'acquisition et d'enregistrerment, et déclencher l'événement utilisateur pour arrêter la boucle de gestion d'événements."
        n93 = Variant To Data(type=errorcluster {"status"=FALSE, "code"=0, "source"=""} ("error constant"), Variant=w293) -> (data=w292:errorcluster)  [unwired: 1 in, 1 out]
        n94 = call <vilib>:"Simple Error Handler.vi"("error in (no error)"=w292) -> ()  [unwired: 4 in, 5 out]
        n95 = call-poly "Enqueue Message.vi"("Message prioritaire ? (F)"=w297, "error in (no error)"=w295, "Message"=w298, "File d'attente de messages"=w302) -> ("error out"=w299:T8)  [unwired: 6 in, 1 out]
        n96 = call-poly "Enqueue Message.vi"("Message prioritaire ? (F)"=w297, "error in (no error)"=w299, "Message"=w298, "File d'attente de messages"=w301) -> ("error out"=w296:T8)  [unwired: 6 in, 1 out]
        n97 = call "Fire User Event - Stop.vi"("error in (no error)"=w296, "Événement utilisateur - Arrêt"=w306) -> ("error out"=w305:T8)  [unwired: 9 in]
      }
      frame "---Copy This Frame---" {
        # "Dupliquez cette étape pour créer de nouveaux messages.  Changez ce commentaire dans l'étape dupliquée pour décrire ce message."
        n98 = Merge Errors(w312) -> (w311:errorcluster)
      }
      frame "Status des paramètres" {
        # "Dupliquez cette étape pour créer de nouveaux messages.  Changez ce commentaire dans l'étape dupliquée pour décrire ce message."
        n99 = Unbundle By Name(w316) -> ("Mode de longueur d'onde.Choix du mode"=w315:bool, "Mode de longueur d'onde.Commande numérique"=w314:dbl)
        n100 = case shown="Vrai" w315 {
          tunnel: [w323 w328] -> w313
          tunnel: w314 -> [_ w329]
          frame False {
            n101 = Concatenate Strings ("Concaténer des chaînes")("Status: Mode automatique") -> (w323:string)
          }
          frame True {
            n102 = Number To Decimal String(number=w329) -> (decimal integer string=w326:string)  [unwired: 1 in]
            n103 = Concatenate Strings ("Concaténer des chaînes")("Status: Mode manuel et la longueur d'onde sélectionnée est ", w326, " nm.") -> (w328:string)
          }
        }
        n104 = Merge Errors(w322) -> (w321:errorcluster)
        n105 = call-poly "Enqueue Message.vi"("Données de message"=w313, "Message"="Update Status", "File d'attente de messages"=w318) -> ()  [unwired: 7 in, 2 out]
      }
      frame Default {
        # "La condition 'Par défaut' ne s'exécute que s'il y a un message qui n'est défini dans aucune des autres conditions.  Renvoyer une erreur de programmation."
        n106 = xnode ("Error Ring")("paramètre 0"=w331) -> ("sortie d'erreur"=w330:errorcluster)
      }
    }
    n107 = call "Error Handler - Message Handling Loop.vi"("error in (no error)"=w77, "File d'attente de messages"=w76) -> ("erreur en entrée dup."=w78:T8)  [unwired: 8 in, 1 out]
  }
  n108 = Unregister For Events(event registration refnum=w19, error in=w26) -> (error out=w20:errorcluster)
  n109 = Release Queue(queue=w14, error in (no error)=w27) -> (error out=w12:errorcluster)  [unwired: 1 in, 2 out]
  n110 = Release Queue(queue=w9, error in (no error)=w12) -> (error out=w11:errorcluster)  [unwired: 1 in, 2 out]
  n111 = Release Notifier(notifier=w8, error in (no error)=w11) -> (error out=w10:errorcluster)  [unwired: 1 in, 2 out]
  n112 = Merge Errors(w20, w10, w25, w22) -> (w15:errorcluster)
  n113 = call "Destroy User Event - Stop.vi"("error in (no error)"=w15, "Événement utilisateur - Arrêt"=w3) -> ("error out"=w13:T8)  [unwired: 9 in]
  n114 = disable-structure "Conditional Disable Structure" shown="RUN_TIME_ENGINE==True" {
    disable-tunnel: w13 -> [_ _]
    frame condition #0 (active) {
    }
    frame condition #1 {
      # "Appeler la fonction Quitter LabVIEW si c'est une application construite."
      n115 = Quit LabVIEW() -> ()  [unwired: 1 in]
    }
  }
